vi "variant2Attributes.vi"(0 "HGV_PVBase":refnum<class "HGF_PVBase.lvclass">, 2 "rawData":variant, 3 "typeDescriptor":string, 5 "error in (no error)":errorcluster) -> (14 "HGV_PVBase":refnum<class "HGF_PVBase.lvclass">, 15 "no link":bool, 16 "Parameter":variant, 17 "typeDescriptor":string, 19 "error out":errorcluster)   [LabVIEW 2014, in "HGF_BaseClasses.lvlib" / "HGF_PVBase.lvclass"]
doc: "Convert raw data value of variant to variant attributes Pn, n=0,1,2,..."
uses:
  HGF_PVBase.lvclass
  HGF_PVDataConverter/HGF_PVDataConverter.lvclass
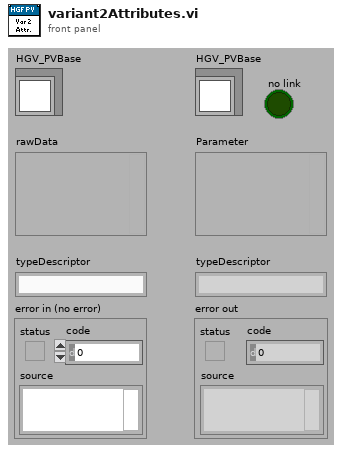
[diagram p1: front panel]
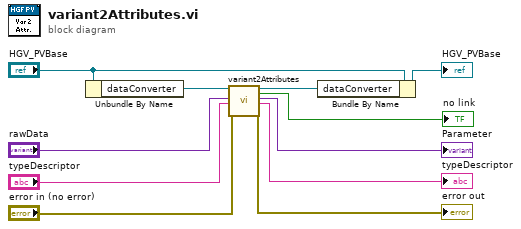
[diagram p0: block diagram]
diagram:
  n1 = Unbundle By Name("HGV_PVBase") -> ("dataConverter"=w11:refnum<class "HGF_PVDataConverter.lvclass">)
  n2 = call-dynamic "variant2Attributes.vi"("HGF_PVDataConverter"=w11, "rawData"="rawData", "typeDescriptor"="typeDescriptor", "error in (no error)"="error in (no error)") -> ("HGF_PVDataConverter"=w8:refnum<class "HGF_PVDataConverter.lvclass">, "no link"=→"no link":bool, "Parameter"=→"Parameter":variant, "typeDescriptor"=→"typeDescriptor":string, "error out"=→"error out":errorcluster)  [unwired: 11 out]
  n3 = Bundle By Name(cluster="HGV_PVBase", "dataConverter"=w8) -> (→"HGV_PVBase":refnum<class "HGF_PVBase.lvclass">)
